vi "PRO_CheckATP.vi"(7 "ATP Check":bool, 8 "Results IN":T1 {"Resistor 2" format="%.1f"; "Drain" format="%.3f"; "Resistor" format="%.1f"; "Fill" format="%.3f"}, 9 "Switched In":bool, 10 "Inputs":cluster{" Ohms":dbl, "Level OUt":dbl}={" Ohms"=101.0, "Level OUt"=8.030499999999925}, 11 "ChA Spec RNG In":T5={"Specs"=[8.5, 8.5, 7.425, 102.0, 98.0, 102.0, 98.0], "LUT Status"={"ChA/!ChB"=FALSE, "Drain/!Fill"=TRUE, "In Range?"=TRUE, "Switch Range?"=FALSE, "Measure R?"=TRUE, "Vaild R?"=TRUE, "Index(n)"=0, "Index(n)-1"=1, "Index Max"=13, "Index(n-1)"=0}}) -> (0 "Results Out":T1 {"Resistor 2" format="%.1f"; "Drain" format="%.3f"; "Resistor" format="%.1f"; "Fill" format="%.3f"}, 1 "Level Out":T4={"Switched"=FALSE, "Level OUt"=8.030499999999925, "Double Err"=FALSE}, 2 "Err Num":i32, 3 "ChA Spec RNG Out":T5={"Specs"=[8.5, 8.5, 7.425, 102.0, 98.0, 102.0, 98.0], "LUT Status"={"ChA/!ChB"=FALSE, "Drain/!Fill"=TRUE, "In Range?"=TRUE, "Switch Range?"=FALSE, "Measure R?"=TRUE, "Vaild R?"=TRUE, "Index(n)"=0, "Index(n)-1"=1, "Index Max"=13, "Index(n-1)"=0}}, 5 "Switched Out":bool)   [LabVIEW 2024]
uses:
  Control Definitions/Def Spec RNG.ctl
  Control Definitions/Ded LUT_Status.ctl
  Control Definitions/Def_LevelSwitched.ctl
  Control Definitions/DEF_Results1D.ctl
  Control Definitions/DEF_ Results3.ctl
  Control Definitions/Def_ATPStatus.ctl
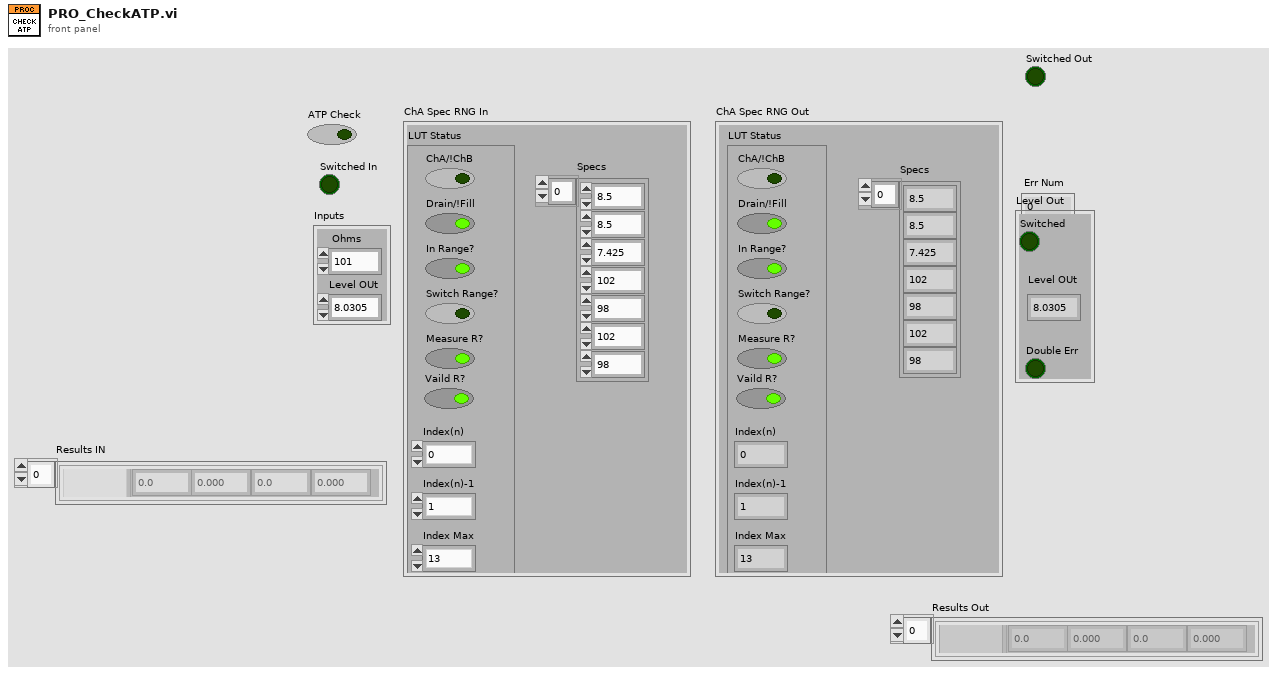
[diagram p1: front panel]
types:
  T1 = typedef "DEF_Results1D.ctl" = T2[]
  T2 = typedef "DEF_ Results3.ctl" = cluster{"Fill":dbl, "Status":T3, "Resistor":dbl, "Drain":dbl, "Resistor 2":dbl}
  T3 = typedef "Def_ATPStatus.ctl" = i16
  T4 = typedef "Def_LevelSwitched.ctl" = cluster{"Switched":bool, "Level OUt":dbl, "Double Err":bool}
  T5 = typedef "Def Spec RNG.ctl" = cluster{"Specs":dbl[], "LUT Status":T6}
  T6 = typedef "Ded LUT_Status.ctl" = cluster{"ChA/!ChB":bool, "Drain/!Fill":bool, "In Range?":bool, "Switch Range?":bool, "Measure R?":bool, "Vaild R?":bool, "Index(n)":i32, "Index(n)-1":i32, "Index Max":i32, "Index(n-1)":i32}
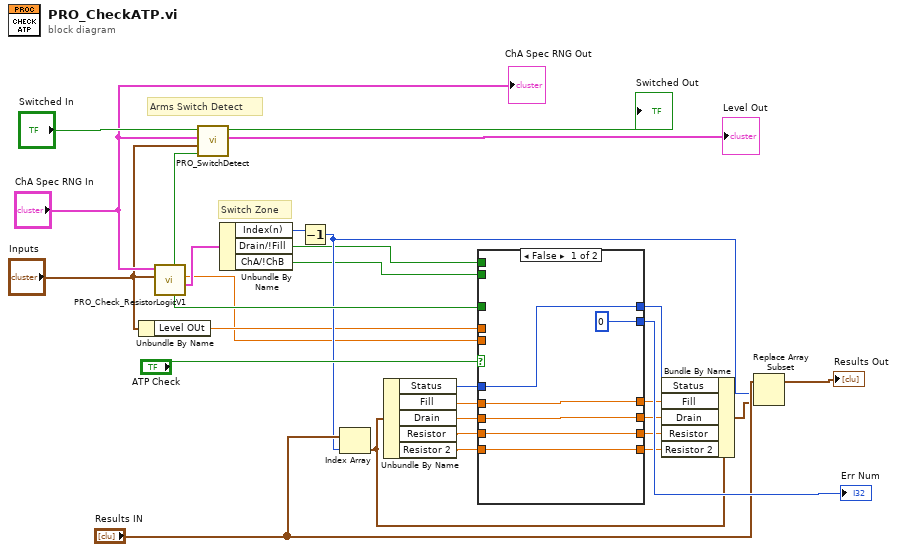
[diagram p0: block diagram]
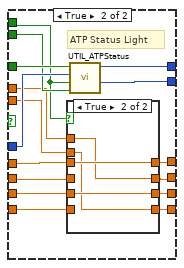
[diagram p2: hidden frame]
diagram:
  # "Switch Zone"
  # "Arms Switch Detect"
  n1 = Unbundle By Name("Inputs") -> ("Level OUt"=w6:dbl)
  n2 = call "PRO_Check_ResistorLogicV1.vi"("Inputs"="Inputs", "ChA Spec RNG In"="ChA Spec RNG In") -> ("LUT Status"=w26:T6, "Resist Measured"=w1:dbl, "Resist in Spec"=w29:bool, "SwP Threshold?"=w23:bool)  [unwired: 4 in, 2 out]
  n3 = call "PRO_SwitchDetect.vi"("SwP Threshold?"=w23, "Inputs"="Inputs", "ChA Spec RNG In"="ChA Spec RNG In", "Switched In"="Switched In") -> ("Level Out Def out"=→"Level Out":T4, "Switched Out"=→"Switched Out":bool)  [unwired: 6 in]
  n4 = Unbundle By Name(w26) -> ("Index(n)"=w15:i32, "Drain/!Fill"=w13:bool, "ChA/!ChB"=w12:bool)
  n5 = Decrement(x=w15) -> (x-1=w14:i32)
  n6 = Index Array(array="Results IN", index=w14) -> (element=w18:T2)
  n7 = Unbundle By Name(w18) -> ("Status"=w17:T3, "Fill"=w11:dbl, "Drain"=w9:dbl, "Resistor"=w4:dbl, "Resistor 2"=w2:dbl)
  n8 = case shown="False" "ATP Check" {
    tunnel: [w36 w50] -> w16
    tunnel: w17 -> [w36 w51]
    tunnel: w29 -> [_ w52]
    tunnel: [u32 0 ("Err Num") w49] -> w30
    tunnel: w13 -> [_ w42]
    tunnel: w12 -> [_ w48]
    tunnel: w11 -> [w34 w46]
    tunnel: [w34 w47] -> w10
    tunnel: w9 -> [w33 w44]
    tunnel: [w33 w45] -> w8
    tunnel: w6 -> [_ w43]
    tunnel: [w32 w41] -> w5
    tunnel: w4 -> [w32 w40]
    tunnel: [w31 w39] -> w3
    tunnel: w2 -> [w31 w38]
    tunnel: w1 -> [_ w37]
    frame False {
    }
    frame True {
      # "ATP Status Light"
      n9 = case shown="True" w42 {
        tunnel: [w55 w60] -> w47
        tunnel: w46 -> [_ w60]
        tunnel: [w56 w59] -> w45
        tunnel: w44 -> [w56 _]
        tunnel: w43 -> [w55 w59]
        tunnel: [w53 w58] -> w41
        tunnel: w40 -> [_ w58]
        tunnel: [w54 w57] -> w39
        tunnel: w38 -> [w54 _]
        tunnel: w37 -> [w53 w57]
        frame False {
        }
        frame True {
        }
      }
      n10 = call "UTIL_ATPStatus.vi"("ChB!ChA"=w48, "Drain!Fill"=w42, "Status In in"=w51, "Good!Bad"=w52) -> ("Err Num"=w49:u32, "Status In out"=w50:u32)  [unwired: 5 in, 1 out]
    }
  }
  "Err Num" <- w30
  n11 = Bundle By Name(cluster=w18, "Status"=w16, "Fill"=w10, "Drain"=w8, "Resistor"=w5, "Resistor 2"=w3) -> (w19:T2)
  n12 = Replace Array Subset(array="Results IN", new element=w19, index=w14) -> (→"Results Out":T1)
  "ChA Spec RNG Out" <- "ChA Spec RNG In"
